vi "Get Project Path.vi"(8 "error in (no error)":errorcluster, 11 "Coverage Analyzer Process in":refnum<class "Coverage Analyzer Process.lvclass">) -> (0 "error out":errorcluster, 2 "Path":path, 3 "Coverage Analyzer Process out":refnum<class "Coverage Analyzer Process.lvclass">)   [LabVIEW 2020, in "Coverage Analyzer Process.lvclass"]
uses:
  Coverage Analyzer Process.lvclass
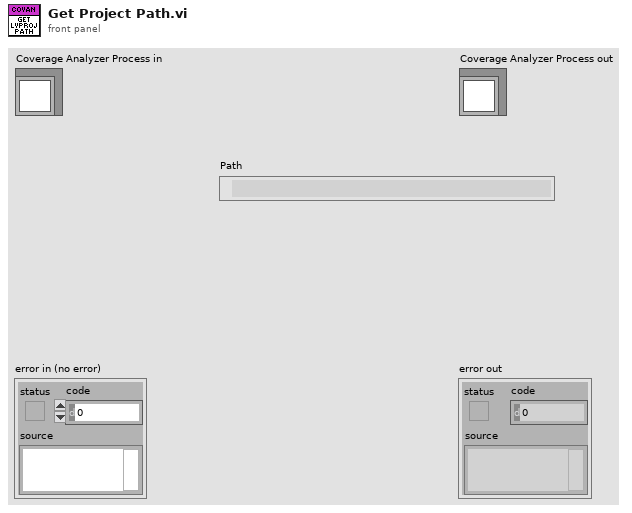
[diagram p1: front panel]
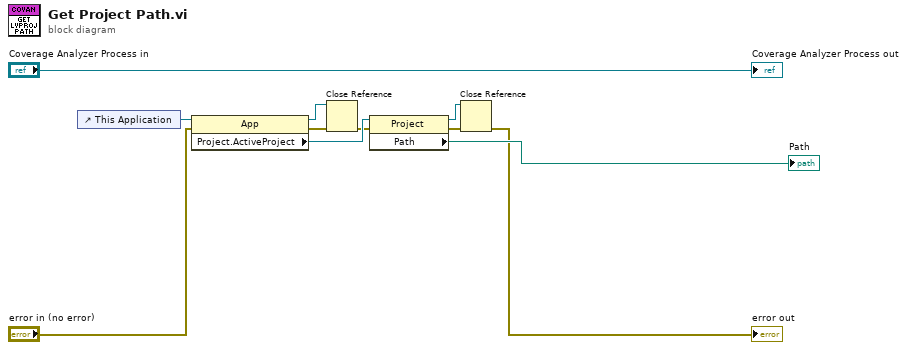
[diagram p0: block diagram]
diagram:
  n1 = control-ref of="This Application"() -> (w10:refnum<vi>)
  n2 = property class="App"(reference=w10, error in="error in (no error)") -> (reference out=w8:refnum<vi>, error out=w5:errorcluster, "Project.ActiveProject"=w9:refnum<vi>)
  n3 = Close Reference(reference=w8, error in (no error)=w5) -> (error out=w4:errorcluster)
  n4 = property class="Project"(reference=w9, error in=w4) -> (reference out=w7:refnum<vi>, error out=w6:errorcluster, "Path"=→"Path":path)
  n5 = Close Reference(reference=w7, error in (no error)=w6) -> (error out=→"error out":errorcluster)
  "Coverage Analyzer Process out" <- "Coverage Analyzer Process in"
